vi "New or Open Excel Workbook.vi"(3 "error in (no error)":errorcluster, 5 "Excel._Application":refnum<k7>) -> (0 "error out":errorcluster, 1 "Excel._Workbooks":refnum<k7>, 2 "Excel._Application":refnum<k7>)   [LabVIEW 2013, in "excel.lvlib"]
uses:
  excel.lvlib
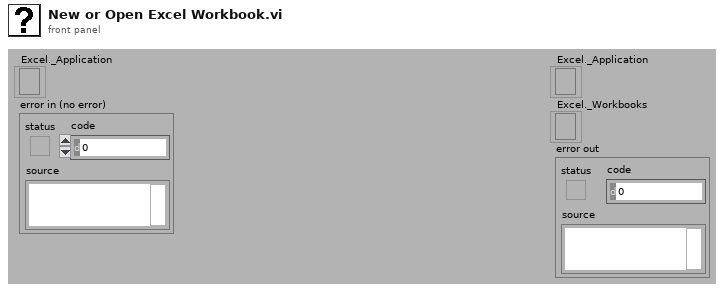
[diagram p1: front panel]
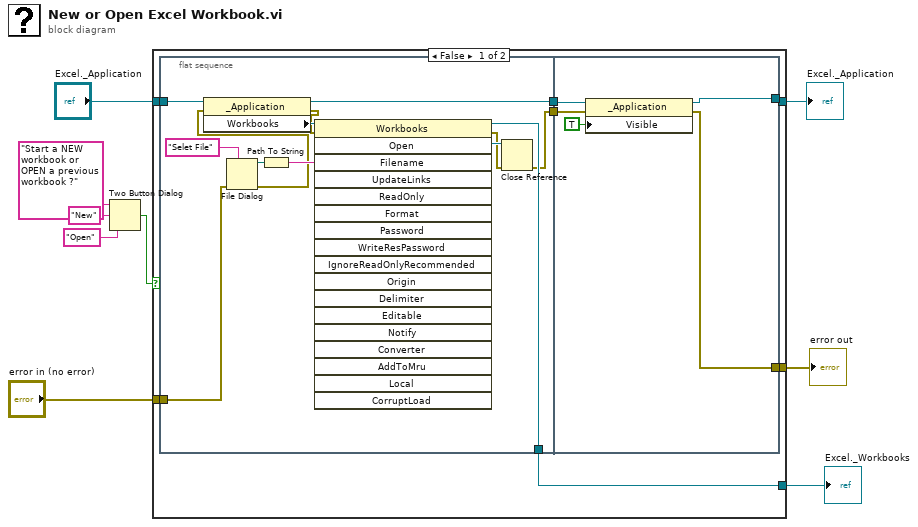
[diagram p0: block diagram]
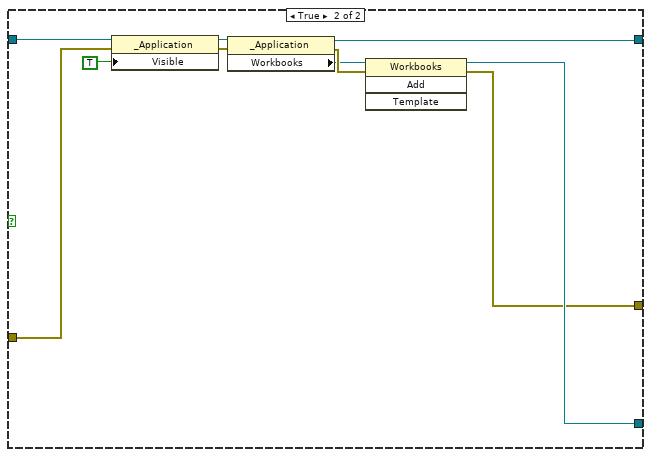
[diagram p2: hidden frame]
diagram:
  n1 = Two Button Dialog(message="Start a NEW workbook or OPEN a previous workbook ?", 1:"Open" ("F button name (\"Cancel\")"), 2:"New" ("T button name (\"OK\")")) -> (T button?=w6:bool)
  n2 = case shown="False" w6 {
    tunnel: "Excel._Application" -> [w16 w40]
    tunnel: [w14 w38] -> w4
    tunnel: [w12 w37] -> w1
    tunnel: "error in (no error)" -> [w10 w36]
    tunnel: [w11 w35] -> w2
    frame False {
      n3 = flat-sequence {
        tunnel: w16 -> [w26]
        tunnel: [w24] -> w15
        tunnel: [w20] -> w13
        tunnel: [w23] -> w12
        tunnel: w10 -> [w17]
        tunnel: w15 -> [w33]
        tunnel: [w32] -> w14
        tunnel: w13 -> [w31]
        tunnel: [w30] -> w11
        frame #0 {
          n4 = File Dialog(7:"Selet File" ("prompt"), 8:w17) -> (0:w18:errorcluster, 3:w28:path)  [unwired: 5 in, 2 out]
          n5 = property class="_Application"(reference=w26, error in=w18) -> (reference out=w24:refnum<k7>, error out=w19:errorcluster, "Workbooks"=w25:refnum<k7>)
          n6 = Path To String(path=w28) -> (string=w29:string)
          n7 = invoke class="Workbooks" method="Open"(reference=w25, error in=w19, "Filename"=w29) -> (reference out=w23:refnum<k7>, error out=w21:errorcluster, "Open"=w22:refnum<k7>)  [unwired: 15 in, 15 out]
          n8 = Close Reference(reference=w22, error in (no error)=w21) -> (error out=w20:errorcluster)
        }
        frame #1 {
          n9 = property class="_Application"(reference=w33, error in=w31, "Visible"=TRUE) -> (reference out=w32:refnum<k7>, error out=w30:errorcluster)
        }
      }
    }
    frame True {
      n10 = property class="_Application"(reference=w40, error in=w36, "Visible"=TRUE) -> (reference out=w41:refnum<k7>, error out=w43:errorcluster)
      n11 = property class="_Application"(reference=w41, error in=w43) -> (reference out=w38:refnum<k7>, error out=w44:errorcluster, "Workbooks"=w42:refnum<k7>)
      n12 = invoke class="Workbooks" method="Add"(reference=w42, error in=w44) -> (reference out=w37:refnum<k7>, error out=w35:errorcluster)  [unwired: 2 in, 2 out]
    }
  }
  "Excel._Application" <- w4
  "Excel._Workbooks" <- w1
  "error out" <- w2
